vi "Remove.vi"(8 "Coords":T1, 11 "Collection In":refnum<class "Collection.lvclass">) -> (3 "Collection Out":refnum<class "Collection.lvclass">)   [LabVIEW 2017, in "Collection.lvclass"]
uses:
  Collection.lvclass
  Coords Cluster.ctl
  Collection.lvclass/Collection.ctl
  Dauntless.lvclass
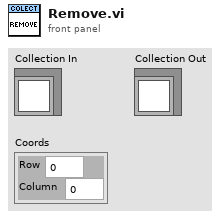
[diagram p1: front panel]
types:
  T1 = typedef "Dauntless.lvclass/Coords Cluster.ctl" = cluster{"Row":i32, "Column":i32}
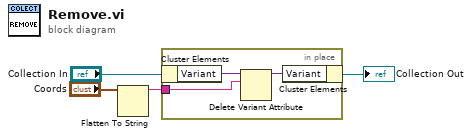
[diagram p0: block diagram]
diagram:
  n1 = Flatten To String(anything="Coords") -> (data string=w1:string)  [unwired: 3 in, 2 out]
  n2 = in-place {
    in-place-border: w1 -> [w6]
    n3 = in-place-cluster #1("Collection In") -> ("Variant"=w7:variant)
    n4 = Delete Variant Attribute(6:w6, 7:w7) -> (3:w5:variant)  [unwired: 1 in, 2 out]
    n5 = in-place-cluster #1("Variant"=w5) -> (→"Collection Out":refnum<class "Collection.lvclass">)
  }
